vi "ke37xx Card Info.vi"(0 "VISA Resource Name":refnum<visa-resource-name>, 7 "Slot":u8=1 min=1 max=6, 11 "error in (no error)":errorcluster) -> (4 "VISA Resource Name Out":refnum<visa-resource-name>, 6 "Card Identification":string, 8 "Card Capabilities":T1, 15 "error out":errorcluster)   [LabVIEW 2009, in "Keithley 3700 Series.lvlib"]
doc: "This VI queries a wide range of card information parameters from a card in a specified slot."
uses:
  <instrlib>/Keithley 3706/Keithley 3700 Series.lvlib
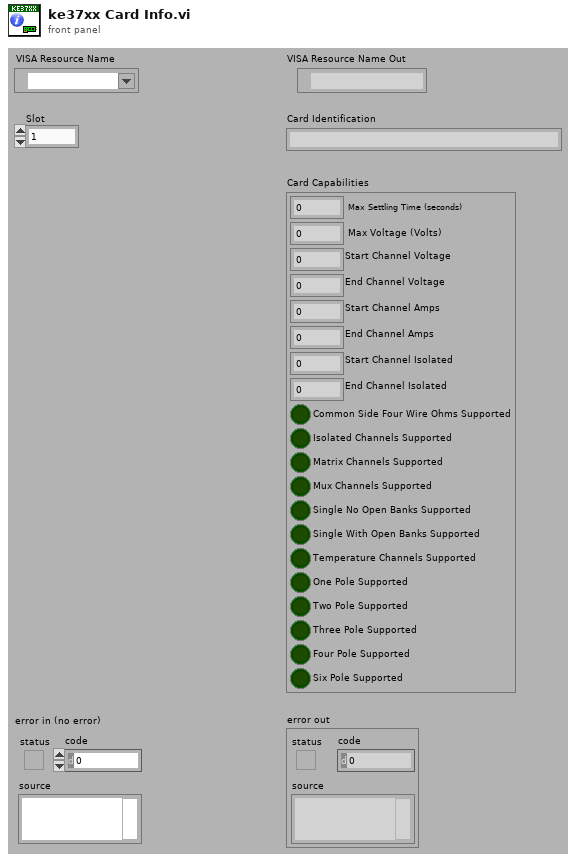
[diagram p1: front panel]
types:
  T1 = cluster{"Max Settling Time (seconds)":dbl, "Max Voltage (Volts)":dbl, "Start Channel Voltage":dbl, "End Channel Voltage":u16, "Start Channel Amps":dbl, "End Channel Amps":dbl, "Start Channel Isolated":dbl, "End Channel Isolated":dbl, "Common Side Four Wire Ohms Supported":bool, "Isolated Channels Supported":bool, "Matrix Channels Supported":bool, "Mux Channels Supported":bool, "Single No Open Banks Supported":bool, "Single With Open Banks Supported":bool, "Temperature Channels Supported":bool, "One Pole Supported":bool, "Two Pole Supported":bool, "Three Pole Supported":bool, "Four Pole Supported":bool, "Six Pole Supported":bool}
  T2 = cluster{"[0]":u16, "[1]":u16, "[2]":u16, "[3]":u16, "[4]":u16, "[5]":u16}
  T3 = cluster{"[0]":bool, "[1]":bool, "[2]":bool, "[3]":bool, "[4]":bool, "[5]":bool, "[6]":bool, "[7]":bool, "[8]":bool, "[9]":bool, "[10]":bool, "[11]":bool}
  T4 = cluster{"[0]":dbl, "[1]":dbl, "[0]":u16, "[1]":u16, "[2]":u16, "[3]":u16, "[4]":u16, "[5]":u16, "[0]":bool, "[1]":bool, "[2]":bool, "[3]":bool, "[4]":bool, "[5]":bool, "[6]":bool, "[7]":bool, "[8]":bool, "[9]":bool, "[10]":bool, "[11]":bool}
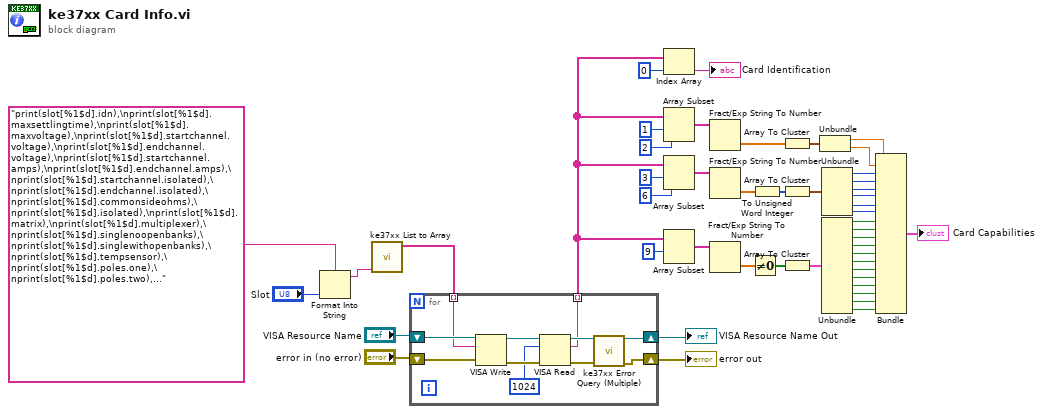
[diagram p0: block diagram]
diagram:
  n1 = Format Into String(format string="print(slot[%1$d].idn),\nprint(slot[%1$d].maxsettlingtime),\nprint(slot[%1$d].maxvoltage),\nprint(slot[%1$d].startchannel.voltage),\nprint(slot[%1$d].endchannel.voltage),\nprint(slot[%1$d].startchannel.amps),\nprint(slot[%1$d].endchannel.amps),\nprint(slot[%1$d].startchannel.isolated),\nprint(slot[%1$d].endchannel.isolated),\nprint(slot[%1$d].commonsideohms),\nprint(slot[%1$d].isolated),\nprint(slot[%1$d].matrix),\nprint(slot[%1$d].multiplexer),\nprint(slot[%1$d].singlenoopenbanks),\nprint(slot[%1$d].singlewithopenbanks),\nprint(slot[%1$d].tempsensor),\nprint(slot[%1$d].poles.one),\nprint(slot[%1$d].poles.two),\nprint(slot[%1$d].poles.three),\nprint(slot[%1$d].poles.four),\nprint(slot[%1$d].poles.six)" ("multi-line string"), "Slot") -> (resulting string=w23:string)  [unwired: 2 in, 1 out]
  n2 = call <instrlib>:"ke37xx List to Array.vi"("List"=w23) -> ("Output String Array"=w25:string[])  [unwired: 1 in, 5 out]
  n3 = for {
    shift-right: [w56] -> w47
    shift-left: "VISA Resource Name" -> [w52]
    shift-right: [w55] -> w46
    shift-left: "error in (no error)" -> [w50]
    tunnel: [w54] -> w18 mode=indexing
    tunnel: w25 -> [w49] mode=indexing
    n4 = VISA Write(VISA resource name=w52, write buffer=w49, error in (no error)=w50) -> (VISA resource name out=w51:refnum<visa-resource-name>, error out=w59:errorcluster)  [unwired: 1 out]
    n5 = VISA Read(VISA resource name=w51, byte count=u32 1024, error in (no error)=w59) -> (VISA resource name out=w58:refnum<visa-resource-name>, read buffer=w54:string, error out=w57:errorcluster)  [unwired: 1 out]
    n6 = call <instrlib>:"ke37xx Error Query (Multiple).vi"("VISA resource name"=w58, "error in (no error)"=w57) -> ("VISA resource name out"=w56:refnum<visa-resource-name>, "error out"=w55:errorcluster)  [unwired: 12 out]
  }
  "VISA Resource Name Out" <- w47
  "error out" <- w46
  n7 = Index Array(array=w18, index=0) -> (element=→"Card Identification":string)
  n8 = Array Subset(array=w18, index=1, length=2) -> (w16:string[])
  n9 = Array Subset(array=w18, index=3, length=6) -> (w17:string[])
  n10 = Array Subset(array=w18, index=9) -> (w40:string[])  [unwired: 1 in]
  n11 = Fract/Exp String To Number(string=w16) -> (number=w6:dbl[])  [unwired: 4 out]
  n12 = Fract/Exp String To Number(string=w17) -> (number=w15:dbl[])  [unwired: 4 out]
  n13 = Fract/Exp String To Number(string=w40) -> (number=w42:dbl[])  [unwired: 4 out]
  n14 = Not Equal To 0?(x=w42) -> (x != 0?=w43:bool[])
  n15 = To Unsigned Word Integer(number=w15) -> (unsigned 16bit integer=w13:u16[])
  n16 = Array To Cluster(array=w6) -> (cluster=w5:cluster{"[0]":dbl, "[1]":dbl})
  n17 = Array To Cluster(array=w13) -> (cluster=w14:T2)
  n18 = Array To Cluster(array=w43) -> (cluster=w39:T3)
  n19 = Unbundle(w5) -> ("[0]"=w3:dbl, "[1]"=w4:dbl)
  n20 = Unbundle(w14) -> ("[0]"=w7:u16, "[1]"=w8:u16, "[2]"=w9:u16, "[3]"=w10:u16, "[4]"=w11:u16, "[5]"=w12:u16)
  n21 = Unbundle(w39) -> ("[0]"=w27:bool, "[1]"=w28:bool, "[2]"=w29:bool, "[3]"=w30:bool, "[4]"=w31:bool, "[5]"=w32:bool, "[6]"=w33:bool, "[7]"=w34:bool, "[8]"=w35:bool, "[9]"=w36:bool, "[10]"=w37:bool, "[11]"=w38:bool)
  n22 = Bundle("[0]"=w3, "[1]"=w4, "[0]"=w7, "[1]"=w8, "[2]"=w9, "[3]"=w10, "[4]"=w11, "[5]"=w12, "[0]"=w27, "[1]"=w28, "[2]"=w29, "[3]"=w30, "[4]"=w31, "[5]"=w32, "[6]"=w33, "[7]"=w34, "[8]"=w35, "[9]"=w36, "[10]"=w37, "[11]"=w38) -> (→"Card Capabilities":T4)  [unwired: 1 out]
